vi "Example One Stage_Patrick_JKISM.vi"() -> ()   [LabVIEW 2019]
uses:
  <userlib>/LevyLab/Xeryon-Rotator/lvsrc/drivers/Class/Controller/Controller.lvclass
panel:
  out "Current State":string
  in  "Controller":refnum<class "Controller.lvclass">
  in  "STOP":bool
  out "Desired Position\n[selected units]":dbl
  out "Encoder position \n[selected units]":dbl
  in  "Tab Control":enum32{"Motion", "Settings"}(tab)
  in  "gotodesired":bool
  in  "Zero Output":bool
  in  "Go to Home":bool
  in  "Scan Right":bool
  in  "Scan Left":bool
  in  "Continue":bool
  in  "Stop":bool
  in  "Make Step Right":bool
  in  "Step Size \n[selected units]":dbl=1.0 format="%#.2f"
  in  "Make Step Left":bool
  in  "Desired Speed \n[1µm/s or 0,01deg /s]":dbl=10000.0 format="%#.2f"
  in  "Desired Position \n[selected units]":dbl format="%#.2f"
  in  "Find Index":bool
  in  "Reset":bool
  out "error out":errorcluster
  in  "Working Units":string(combo)="1000000,0"
  out "StatusBits":T1
  out "Status Info":T2
  in  "Axis Resolution":string(combo)="3.49065850399"
  in  "Axis Letter":string="X"
  in  "Baudrate":dbl=9600.0
  in  "COM Port":refnum<visa-resource-name>="COM4"
  out "Waveform Chart":T3(graph)
  in  "STOP PROGRAM":bool
  # "Visualization"
  # "Extra information"
  # "READ ME FIRST"
  # "Configuration"
  # "Stage 1"
  # "Driver 1"
  # "Stage 1"
  # "How to run:"
  # "BEFORE RUNNING:"
  # "1, Select COM Port"
  # "2. Select baudrate"
  # "3. For each axis:"
  # "3.1 Specify correct axis name (1 letter)"
  # "3.2 Specify correct resolution"
  # "4. Run VI"
  # "WHEN RUNNING, YOU HAVE TO FIRST PUSH \"FIND INDEX\" FOR EACH STAGE.\nThe stages will start moving and find its position. After that you can control the stages"
  # "NOTES: Do this only the first time"
  # "3.49065850399"
  # "1. Replace the settings_default.txt file with\nthe file we provided on a USB stick."
  # "2.    Make sure there are no comments in the\nsettings_default.txt file. ONLY lines like: \"X:DPOS=100\" so NO \"%\" in front or at the end of the line."
  # "Position Information"
  # "STOP BUTTON"
  # "3.  In your settings_default.txt file:\nEvery line that contains SSPD or MSPD: multiply that value with:\n - 1000 for a lineair stage \n - 100 for a rotating stage"
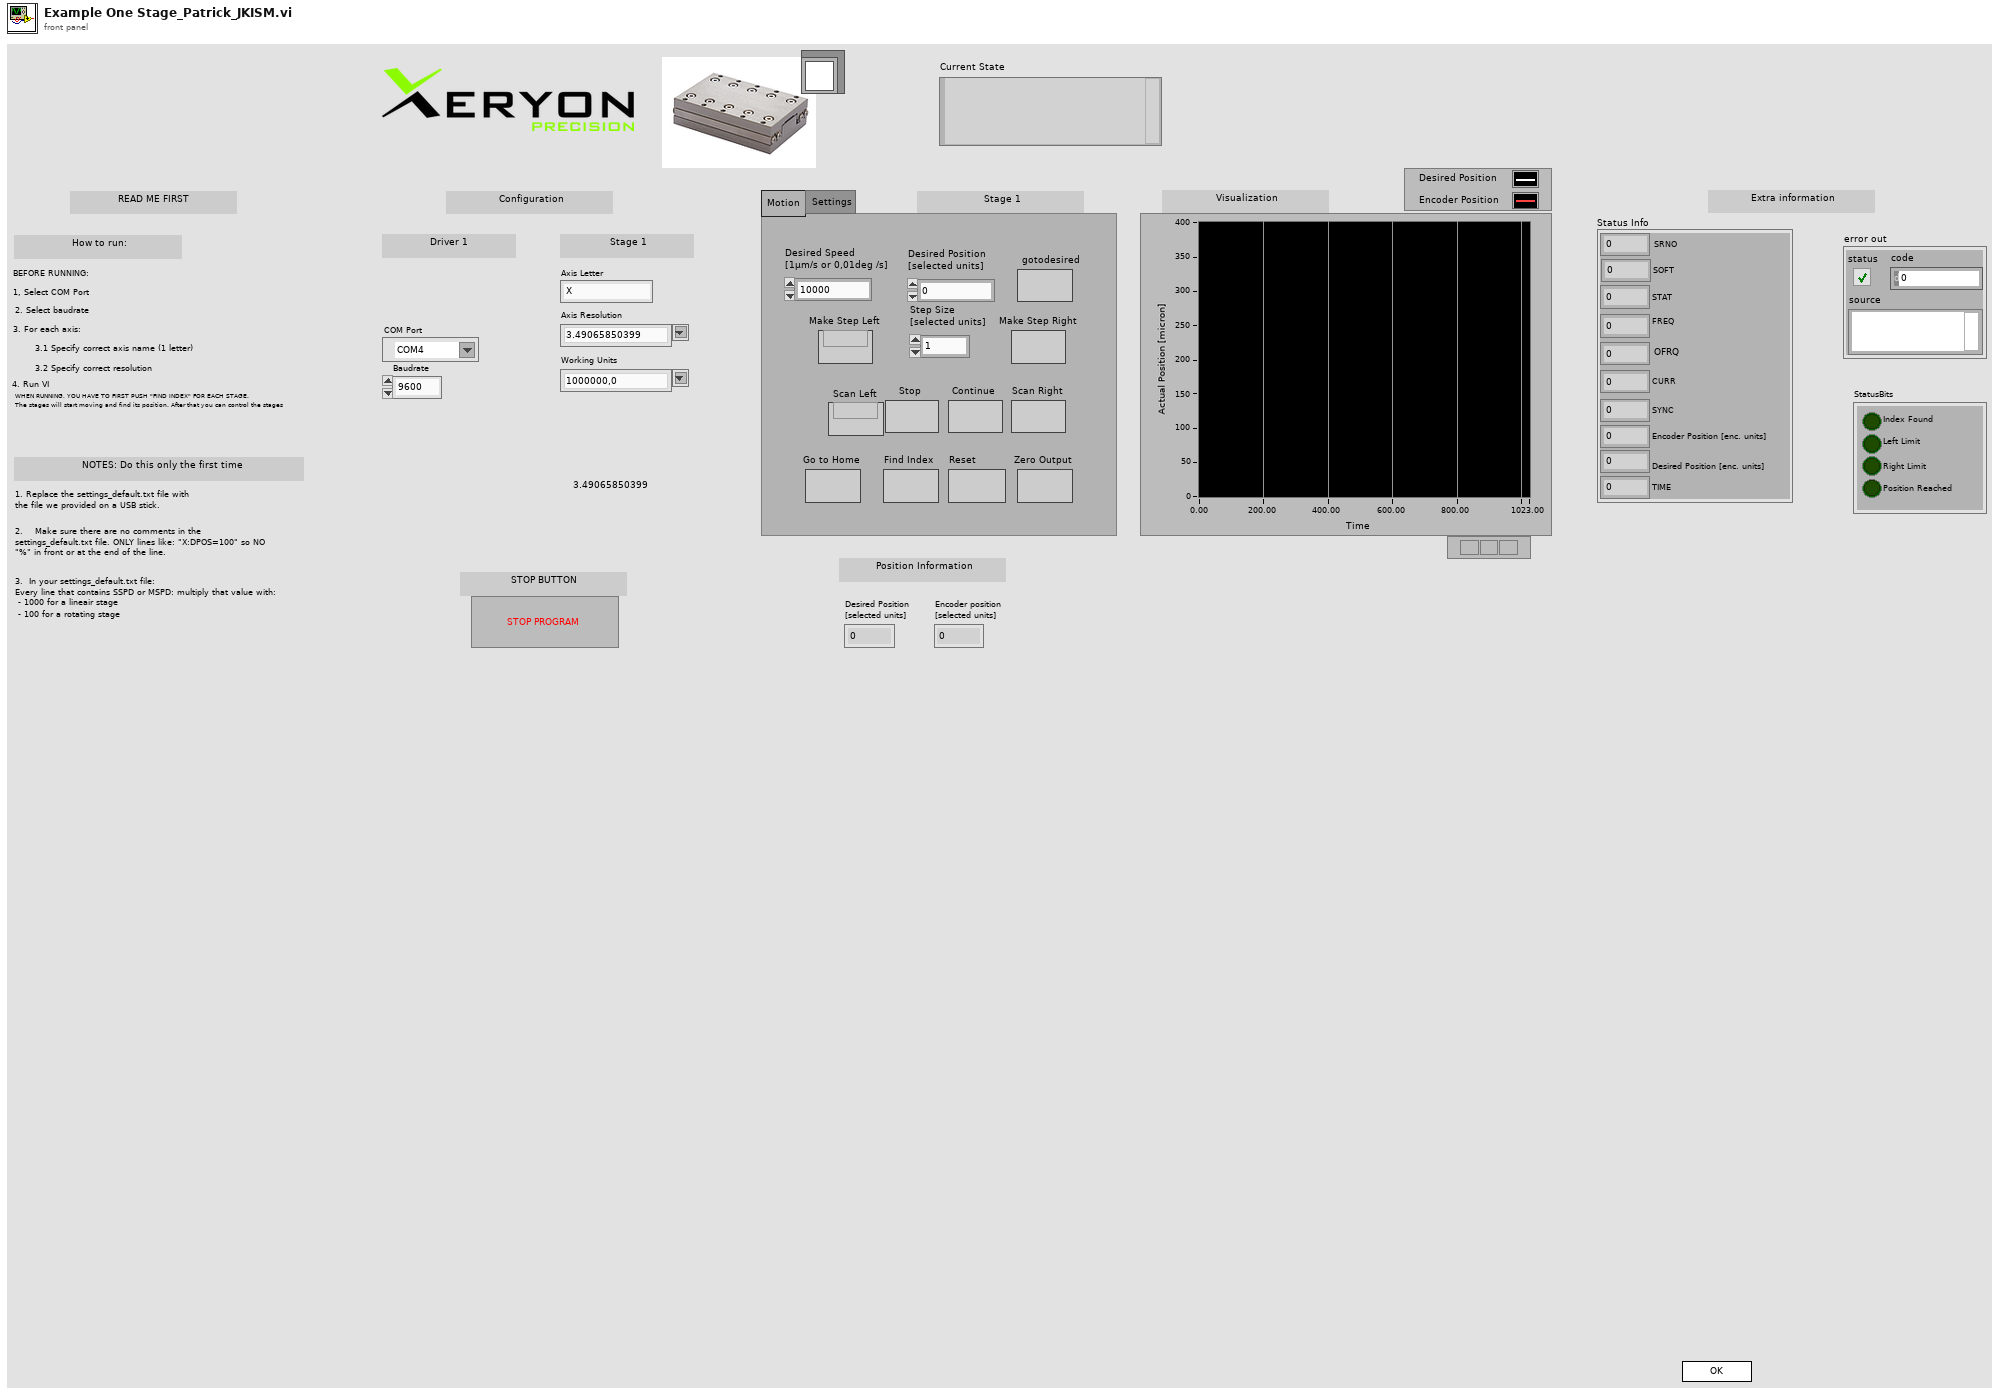
[diagram p1: front panel]
types:
  T1 = cluster{"Index Found":bool, "Left Limit":bool, "Right Limit":bool, "Position Reached":bool}
  T2 = cluster{"SRNO":dbl, "SOFT":dbl, "STAT":dbl, "FREQ":dbl, "OFRQ":dbl, "CURR":dbl, "SYNC":dbl, "Encoder Position [enc. units]":dbl, "Desired Position [enc. units]":dbl, "TIME":dbl}
  T3 = cluster{"DPOS In Current Units":dbl, "EPOS In Current Units":dbl}
  T4 = enum32{"Invalid", "Standard", "Closed", "Hidden", "Minimized", "Maximized"}
  T5 = enum32{"invalid app kind", "Development System", "Run Time System", "Student Edition", "Embedded LabVIEW", "Evaluation", "Custom"}
  T6 = cluster{"Core":cluster{"Current VI Reference":refnum<vi>, "Close Panel on Exit?":bool}, "Controller":refnum<class "Controller.lvclass">, "Axis Letter":string}
  T7 = cluster{"Current VI Reference":refnum<vi>, "Close Panel on Exit?":bool}
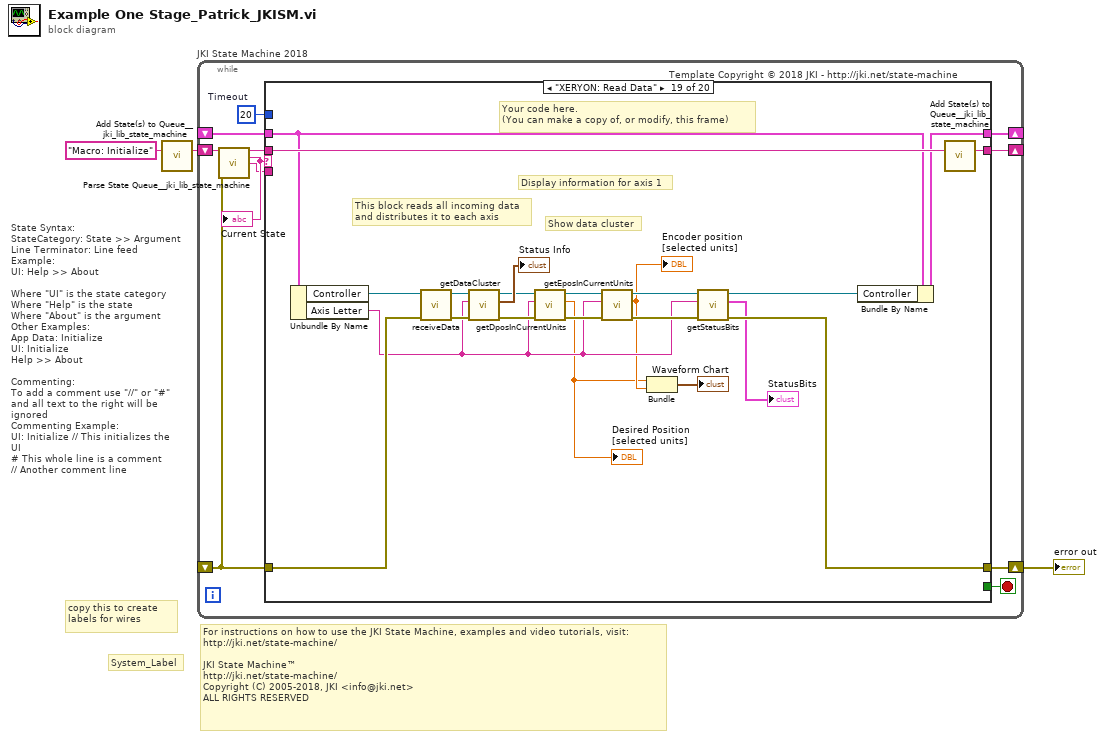
[diagram p0: block diagram]
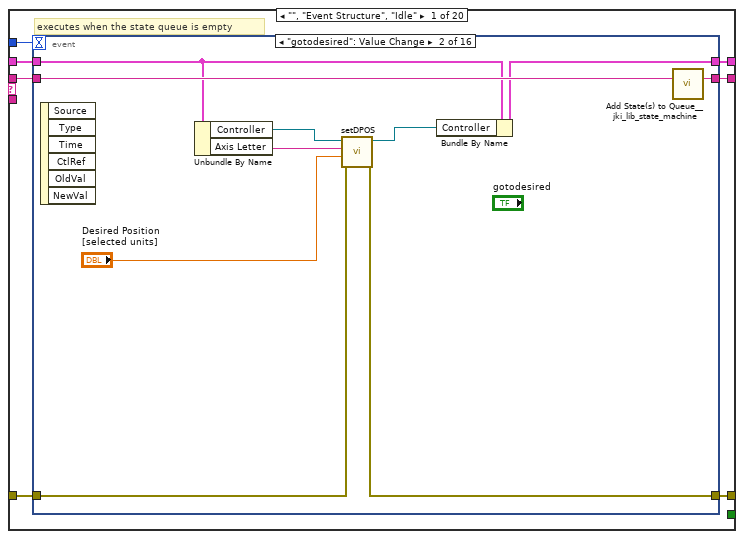
[diagram p2: hidden frame]
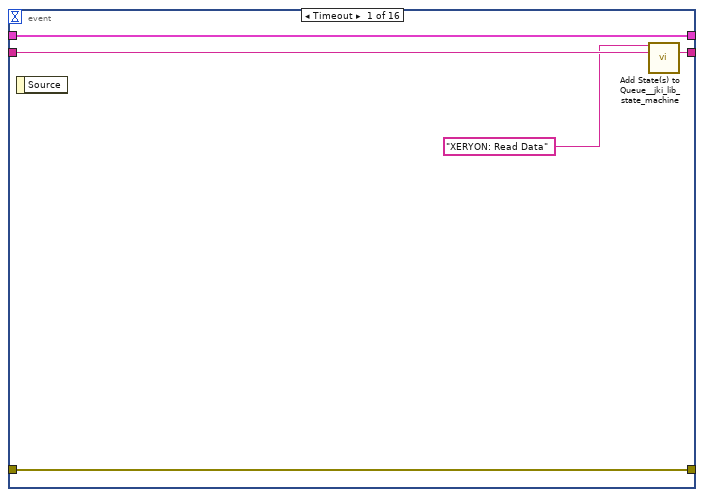
[diagram p3: hidden frame]
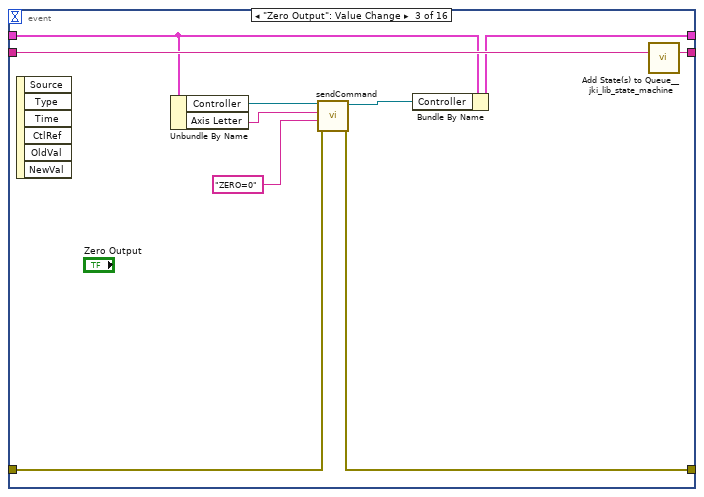
[diagram p4: hidden frame]
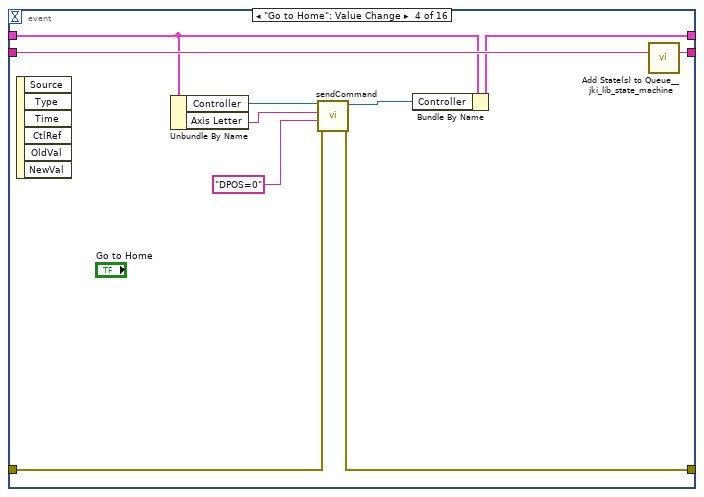
[diagram p5: hidden frame]
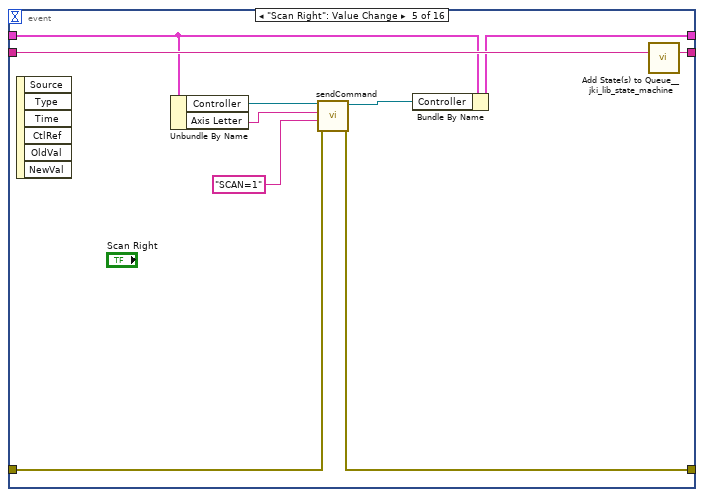
[diagram p6: hidden frame]
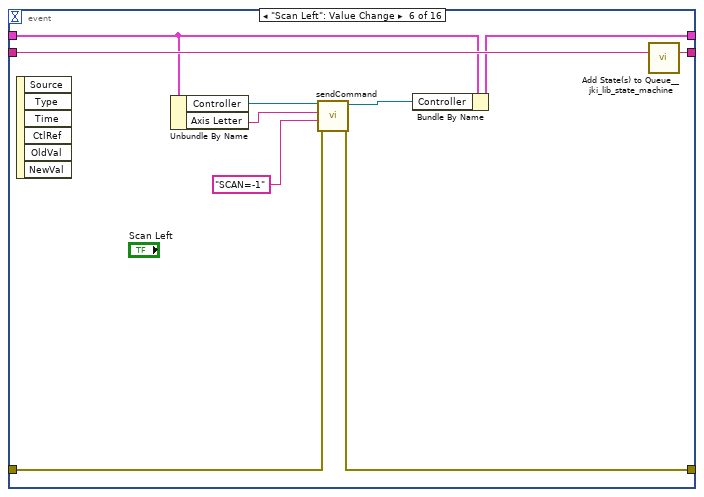
[diagram p7: hidden frame]
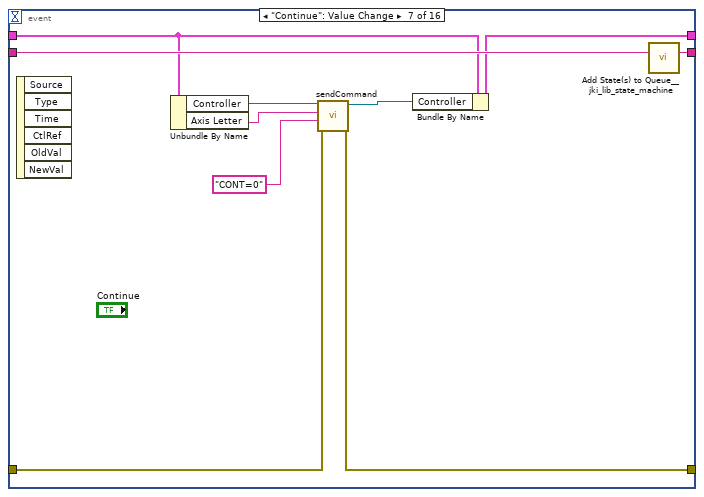
[diagram p8: hidden frame]
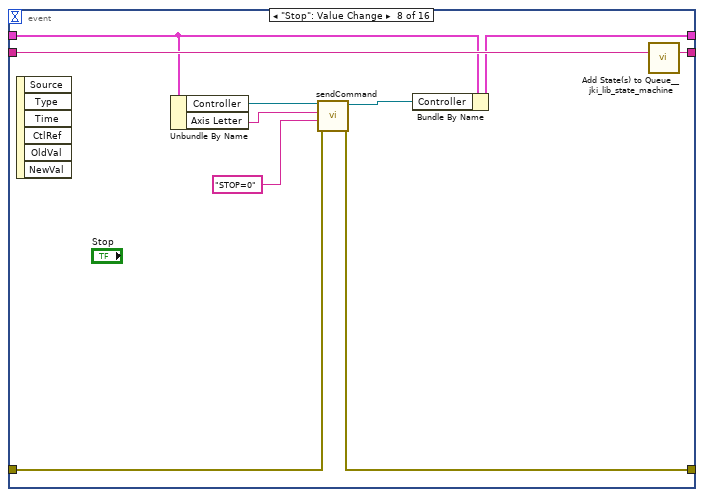
[diagram p9: hidden frame]
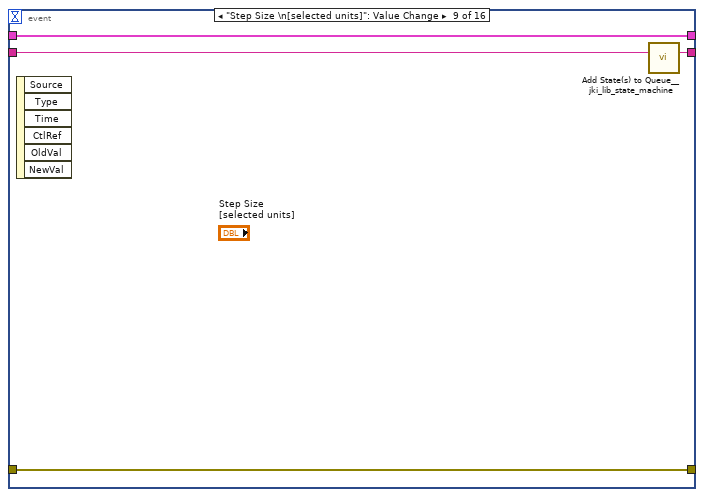
[diagram p10: hidden frame]
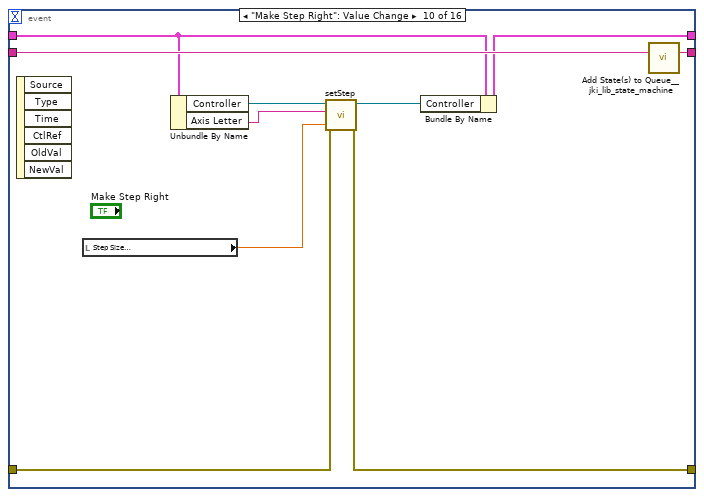
[diagram p11: hidden frame]
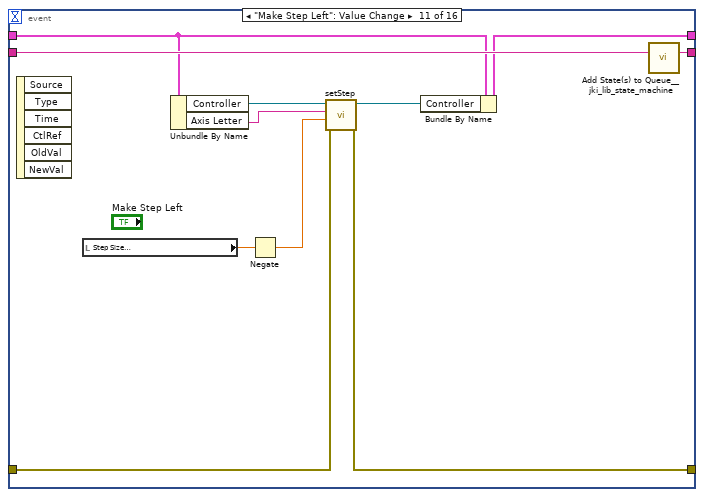
[diagram p12: hidden frame]
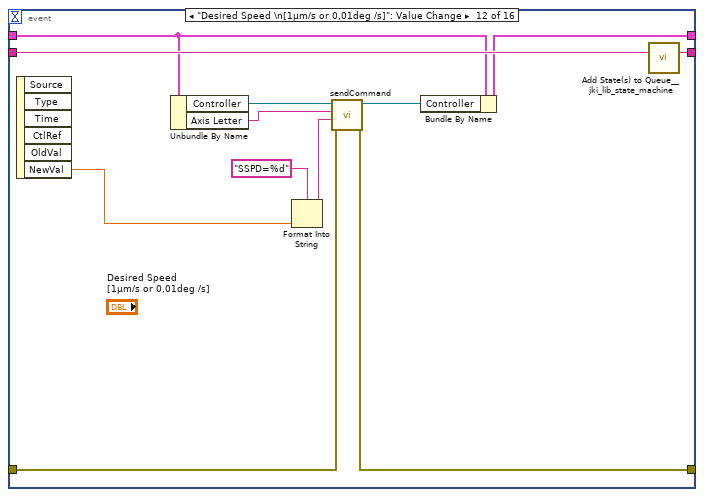
[diagram p13: hidden frame]
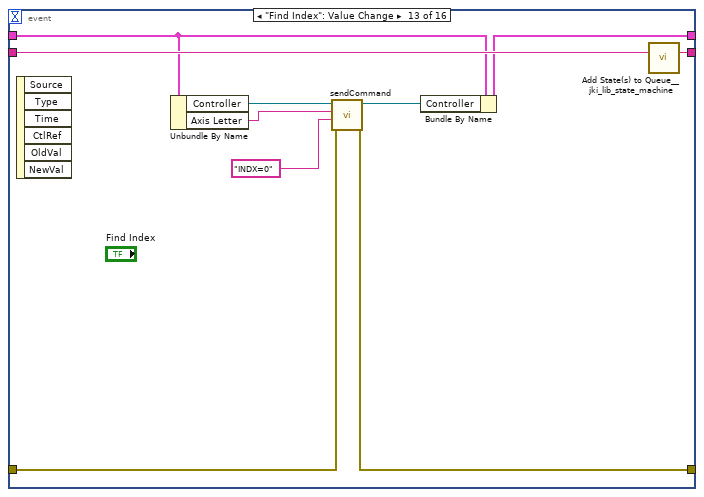
[diagram p14: hidden frame]
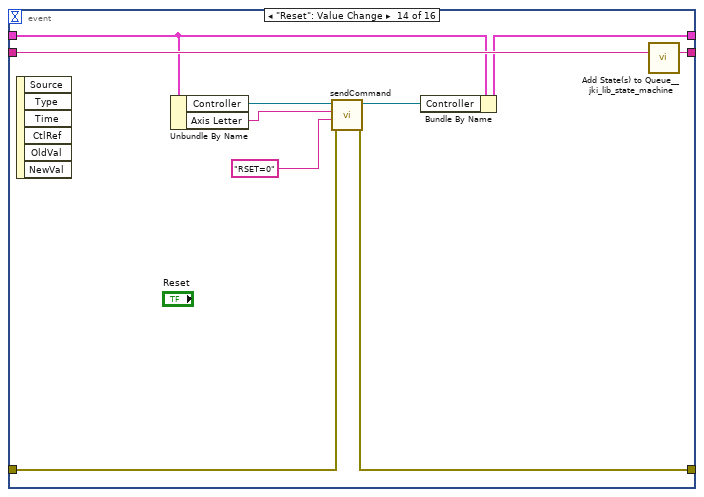
[diagram p15: hidden frame]
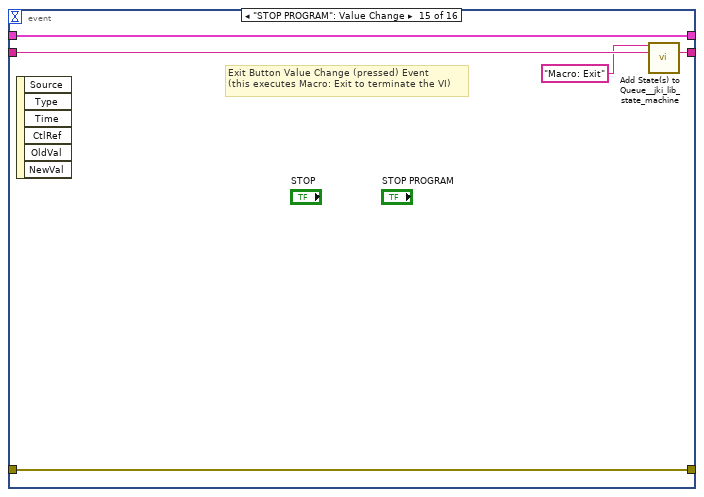
[diagram p16: hidden frame]
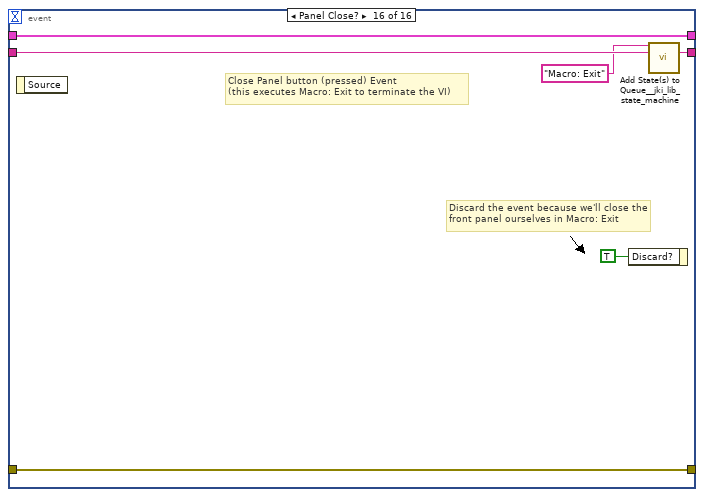
[diagram p17: hidden frame]
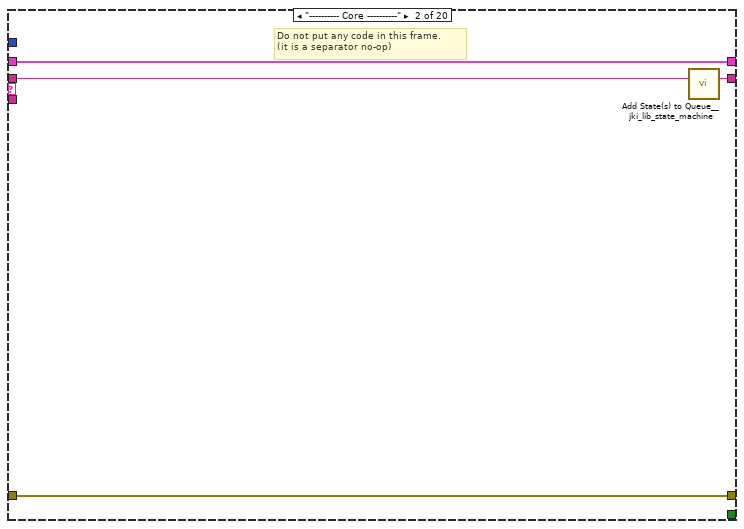
[diagram p18: hidden frame]
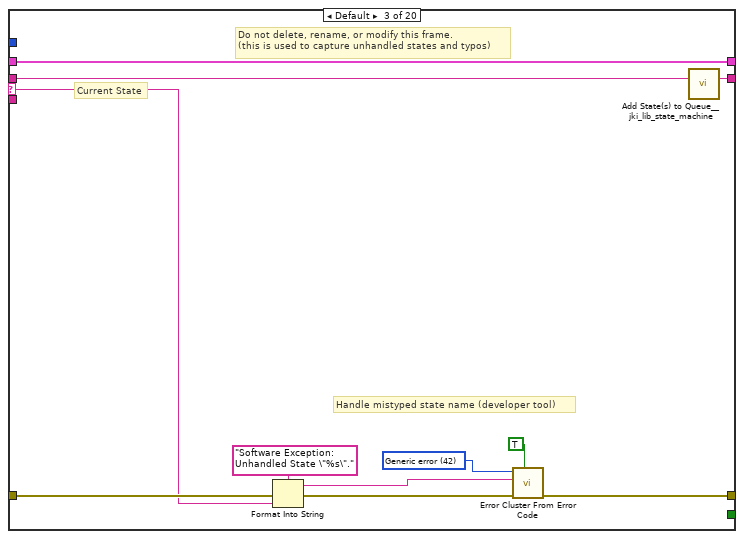
[diagram p19: hidden frame]
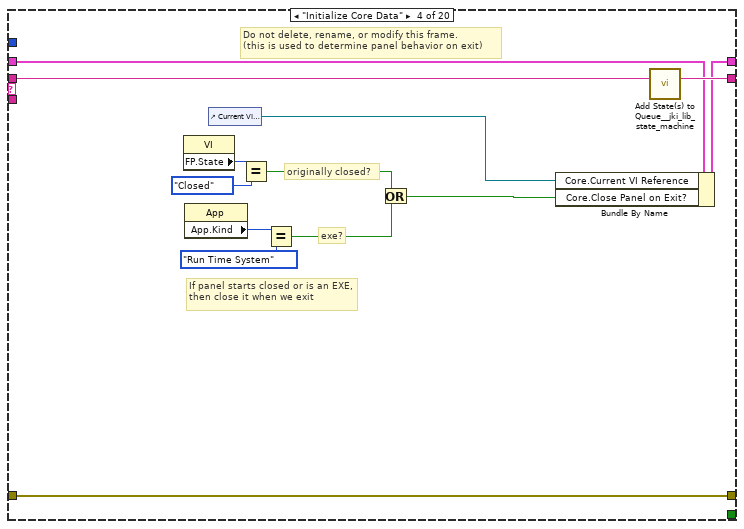
[diagram p20: hidden frame]
diagram:
  # "For instructions on how to use the JKI State Machine, examples and video tutorials, visit:\nhttp://jki.net/state-machine/\n\nJKI State Machine™\nhttp://jki.net/state-machine/\nCopyright (C) 2005-2018, JKI <info@jki.net>\nALL RIGHTS RESERVED"
  # "State Syntax:\nStateCategory: State >> Argument\nLine Terminator: Line feed\nExample:\nUI: Help >> About\n\nWhere \"UI\" is the state category\nWhere \"Help\" is the state\nWhere \"About\" is the argument\nOther Examples:\nApp Data: Initialize\nUI: Initialize\nHelp >> About\n\nCommenting:\nTo add a comment use \"//\" or \"#\" and all text to the right will be ignored\nCommenting Example:\nUI: Initialize // This initializes the UI\n# This whole line is a comment\n// Another comment line"
  # "copy this to create labels for wires"
  # "System_Label"
  n1 = call <vilib>:"Add State(s) to Queue__jki_lib_state_machine.vi"("State(s) in (\"\")"="Macro: Initialize") -> ("States Out"=w3:string)  [unwired: 14 in]
  n2 = while "JKI State Machine 2018" {
    shift-right: [w7] -> _
    shift-left: _ -> [w6]
    shift-right: [w10] -> w1
    shift-left: _ -> [w4]
    shift-right: [w9] -> _
    shift-left: w3 -> [w11]
    stop <- w8 stop-if-true
    w5 = 20  # Timeout
    # "Template Copyright © 2018 JKI - http://jki.net/state-machine"
    n3 = call <vilib>:"Parse State Queue__jki_lib_state_machine.vi"("State Queue"=w11, "Error In (no error)"=w4) -> ("Remaining States"=w13:string, "Current State"=w14:string, "Arguments"=w12:string)  [unwired: 11 in]
    "Current State" <- w14
    n4 = case shown="\"XERYON: Read Data\"" w14 {
      selector: w14 -> [_ _ w169 _ _ _ _ _ _ _ _ _ _ _ _ _ _ _ _ _]
      tunnel: w13 -> [w21 w168 w173 w192 w198 w203 w207 w214 w220 w224 w228 w234 w245 w314 w319 w330 w334 w351 w373 w379]
      tunnel: w12 -> [_ _ _ _ _ _ _ _ _ _ _ w229 w239 _ _ _ _ _ _ _]
      tunnel: w6 -> [w19 w165 w171 w185 w195 w201 w204 _ w215 w221 w226 w232 w241 w311 w316 w327 w331 w338 w356 w377]
      tunnel: [w18 w166 w175 w189 errorcluster {"status"=FALSE, "code"=0, "source"=""} ("error out") w200 w205 w211 w216 w222 w225 w230 w242 w312 w317 w328 w332 w336 w360 w375] -> w10
      tunnel: w4 -> [w17 w166 w174 w189 w194 w200 w205 w211 w217 w222 w225 w231 w243 w312 w317 w328 w332 w335 w359 w374]
      tunnel: [w20 w167 w172 w191 w197 w202 w206 w213 w219 w223 w227 w233 w244 w313 w318 w329 w333 w350 w372 w378] -> w9
      tunnel: [_ _ _ _ _ TRUE _ _ _ _ _ _ _ _ _ _ _ _ _ _] -> w8
      tunnel: [w16 w165 w171 w190 w195 w201 w204 w212 w215 w221 w226 w232 w241 w311 w316 w327 w331 w349 w357 w377] -> w7
      tunnel: w5 -> [w15 _ _ _ _ _ _ _ _ _ _ _ _ _ _ _ _ _ _ _]
      frame "", "Event Structure", "Idle" {
        # "executes when the state queue is empty"
        n5 = event shown="[1] \"gotodesired\": Value Change" {
          selector: _ -> [_ _ _ _ _ _ _ _ _ _ _ _ _ _ _ _]
          dyn-events: _ -> [_ _ _ _ _ _ _ _ _ _ _ _ _ _ _ _]
          timeout: w15 -> [_ _ _ _ _ _ _ _ _ _ _ _ _ _ _ _]
          tunnel: w21 -> [w26 w36 w46 w56 w66 w76 w86 w96 w100 w110 w121 w133 w143 w153 w158 w164]
          tunnel: [w25 w35 w45 w55 w65 w75 w85 w95 w99 w109 w120 w132 w142 w152 w157 w163] -> w20
          tunnel: w19 -> [w23 w30 w43 w53 w63 w73 w83 w93 w98 w107 w118 w130 w140 w150 w155 w161]
          tunnel: [w24 w29 w37 w47 w57 w67 w77 w87 w97 w101 w112 w122 w135 w145 w156 w162] -> w18
          tunnel: w17 -> [w24 w28 w38 w48 w58 w68 w78 w88 w97 w102 w113 w123 w136 w146 w156 w162]
          tunnel: [w23 w31 w44 w54 w64 w74 w84 w94 w98 w108 w119 w131 w141 w151 w155 w161] -> w16
          event Timeout {
            n6 = event-data() -> ()  [unwired: 1 in, 1 out]
            n7 = call <vilib>:"Add State(s) to Queue__jki_lib_state_machine.vi"("State(s) in Front (\"\")"="XERYON: Read Data" ("State(s) in Front (\"\")"), "State(s) in (\"\")"=w26) -> ("States Out"=w25:string)  [unwired: 13 in]
          }
          event "gotodesired": Value Change {
            n8 = event-data() -> ()  [unwired: 1 in, 6 out]
            n9 = Unbundle By Name(w30) -> ("Controller"=w33:refnum<class "Controller.lvclass">, "Axis Letter"=w34:string)
            n10 = call-dynamic "setDPOS.vi"("error in (no error)"=w28, "DPOS In Current Units"="Desired Position \n[selected units]", "Axis Letter"=w34, "Controller in"=w33) -> ("error out"=w29:errorcluster, "Controller out"=w32:refnum<class "Controller.lvclass">)  [unwired: 6 in]
            n11 = Bundle By Name(cluster=w30, "Controller"=w32) -> (w31:T6)
            n12 = call <vilib>:"Add State(s) to Queue__jki_lib_state_machine.vi"("State(s) in (\"\")"=w36) -> ("States Out"=w35:string)  [unwired: 14 in]
          }
          event "Zero Output": Value Change {
            n13 = event-data() -> ()  [unwired: 1 in, 6 out]
            n14 = Unbundle By Name(w43) -> ("Controller"=w41:refnum<class "Controller.lvclass">, "Axis Letter"=w40:string)
            n15 = call-dynamic "sendCommand.vi"("error in (no error)"=w38, "Command"="ZERO=0", "Axis Letter"=w40, "Controller in"=w41) -> ("error out"=w37:errorcluster, "Controller out"=w39:refnum<class "Controller.lvclass">)  [unwired: 6 in]
            n16 = Bundle By Name(cluster=w43, "Controller"=w39) -> (w44:T6)
            n17 = call <vilib>:"Add State(s) to Queue__jki_lib_state_machine.vi"("State(s) in (\"\")"=w46) -> ("States Out"=w45:string)  [unwired: 14 in]
          }
          event "Go to Home": Value Change {
            n18 = event-data() -> ()  [unwired: 1 in, 6 out]
            n19 = Unbundle By Name(w53) -> ("Controller"=w51:refnum<class "Controller.lvclass">, "Axis Letter"=w50:string)
            n20 = call-dynamic "sendCommand.vi"("error in (no error)"=w48, "Command"="DPOS=0", "Axis Letter"=w50, "Controller in"=w51) -> ("error out"=w47:errorcluster, "Controller out"=w49:refnum<class "Controller.lvclass">)  [unwired: 6 in]
            n21 = Bundle By Name(cluster=w53, "Controller"=w49) -> (w54:T6)
            n22 = call <vilib>:"Add State(s) to Queue__jki_lib_state_machine.vi"("State(s) in (\"\")"=w56) -> ("States Out"=w55:string)  [unwired: 14 in]
          }
          event "Scan Right": Value Change {
            n23 = event-data() -> ()  [unwired: 1 in, 6 out]
            n24 = Unbundle By Name(w63) -> ("Controller"=w61:refnum<class "Controller.lvclass">, "Axis Letter"=w60:string)
            n25 = call-dynamic "sendCommand.vi"("error in (no error)"=w58, "Command"="SCAN=1", "Axis Letter"=w60, "Controller in"=w61) -> ("error out"=w57:errorcluster, "Controller out"=w59:refnum<class "Controller.lvclass">)  [unwired: 6 in]
            n26 = Bundle By Name(cluster=w63, "Controller"=w59) -> (w64:T6)
            n27 = call <vilib>:"Add State(s) to Queue__jki_lib_state_machine.vi"("State(s) in (\"\")"=w66) -> ("States Out"=w65:string)  [unwired: 14 in]
          }
          event "Scan Left": Value Change {
            n28 = event-data() -> ()  [unwired: 1 in, 6 out]
            n29 = Unbundle By Name(w73) -> ("Controller"=w71:refnum<class "Controller.lvclass">, "Axis Letter"=w70:string)
            n30 = call-dynamic "sendCommand.vi"("error in (no error)"=w68, "Command"="SCAN=-1", "Axis Letter"=w70, "Controller in"=w71) -> ("error out"=w67:errorcluster, "Controller out"=w69:refnum<class "Controller.lvclass">)  [unwired: 6 in]
            n31 = Bundle By Name(cluster=w73, "Controller"=w69) -> (w74:T6)
            n32 = call <vilib>:"Add State(s) to Queue__jki_lib_state_machine.vi"("State(s) in (\"\")"=w76) -> ("States Out"=w75:string)  [unwired: 14 in]
          }
          event "Continue": Value Change {
            n33 = event-data() -> ()  [unwired: 1 in, 6 out]
            n34 = Unbundle By Name(w83) -> ("Controller"=w81:refnum<class "Controller.lvclass">, "Axis Letter"=w80:string)
            n35 = call-dynamic "sendCommand.vi"("error in (no error)"=w78, "Command"="CONT=0", "Axis Letter"=w80, "Controller in"=w81) -> ("error out"=w77:errorcluster, "Controller out"=w79:refnum<class "Controller.lvclass">)  [unwired: 6 in]
            n36 = Bundle By Name(cluster=w83, "Controller"=w79) -> (w84:T6)
            n37 = call <vilib>:"Add State(s) to Queue__jki_lib_state_machine.vi"("State(s) in (\"\")"=w86) -> ("States Out"=w85:string)  [unwired: 14 in]
          }
          event "Stop": Value Change {
            n38 = event-data() -> ()  [unwired: 1 in, 6 out]
            n39 = Unbundle By Name(w93) -> ("Controller"=w91:refnum<class "Controller.lvclass">, "Axis Letter"=w90:string)
            n40 = call-dynamic "sendCommand.vi"("error in (no error)"=w88, "Command"="STOP=0", "Axis Letter"=w90, "Controller in"=w91) -> ("error out"=w87:errorcluster, "Controller out"=w89:refnum<class "Controller.lvclass">)  [unwired: 6 in]
            n41 = Bundle By Name(cluster=w93, "Controller"=w89) -> (w94:T6)
            n42 = call <vilib>:"Add State(s) to Queue__jki_lib_state_machine.vi"("State(s) in (\"\")"=w96) -> ("States Out"=w95:string)  [unwired: 14 in]
          }
          event "Step Size \n[selected units]": Value Change {
            n43 = event-data() -> ()  [unwired: 1 in, 6 out]
            n44 = call <vilib>:"Add State(s) to Queue__jki_lib_state_machine.vi"("State(s) in (\"\")"=w100) -> ("States Out"=w99:string)  [unwired: 14 in]
          }
          event "Make Step Right": Value Change {
            n45 = event-data() -> ()  [unwired: 1 in, 6 out]
            n46 = local read "Step Size \n[selected units]"() -> (w103:dbl)
            n47 = Unbundle By Name(w107) -> ("Controller"=w106:refnum<class "Controller.lvclass">, "Axis Letter"=w104:string)
            n48 = call-dynamic "setStep.vi"("error in (no error)"=w102, "Step Value"=w103, "Axis Letter"=w104, "Controller in"=w106) -> ("error out"=w101:errorcluster, "Controller out"=w105:refnum<class "Controller.lvclass">)  [unwired: 6 in]
            n49 = Bundle By Name(cluster=w107, "Controller"=w105) -> (w108:T6)
            n50 = call <vilib>:"Add State(s) to Queue__jki_lib_state_machine.vi"("State(s) in (\"\")"=w110) -> ("States Out"=w109:string)  [unwired: 14 in]
          }
          event "Make Step Left": Value Change {
            n51 = event-data() -> ()  [unwired: 1 in, 6 out]
            n52 = local read "Step Size \n[selected units]"() -> (w114:dbl)
            n53 = Unbundle By Name(w118) -> ("Controller"=w117:refnum<class "Controller.lvclass">, "Axis Letter"=w115:string)
            n54 = Negate(x=w114) -> (-x=w111:dbl)
            n55 = call-dynamic "setStep.vi"("error in (no error)"=w113, "Step Value"=w111, "Axis Letter"=w115, "Controller in"=w117) -> ("error out"=w112:errorcluster, "Controller out"=w116:refnum<class "Controller.lvclass">)  [unwired: 6 in]
            n56 = Bundle By Name(cluster=w118, "Controller"=w116) -> (w119:T6)
            n57 = call <vilib>:"Add State(s) to Queue__jki_lib_state_machine.vi"("State(s) in (\"\")"=w121) -> ("States Out"=w120:string)  [unwired: 14 in]
          }
          event "Desired Speed \n[1µm/s or 0,01deg /s]": Value Change {
            n58 = event-data() -> ("NewVal"=w124:dbl)  [unwired: 1 in, 5 out]
            n59 = Unbundle By Name(w130) -> ("Controller"=w127:refnum<class "Controller.lvclass">, "Axis Letter"=w125:string)
            n60 = Format Into String(format string="SSPD=%d", w124) -> (resulting string=w129:string)  [unwired: 2 in, 1 out]
            n61 = call-dynamic "sendCommand.vi"("error in (no error)"=w123, "Command"=w129, "Axis Letter"=w125, "Controller in"=w127) -> ("error out"=w122:errorcluster, "Controller out"=w126:refnum<class "Controller.lvclass">)  [unwired: 6 in]
            n62 = Bundle By Name(cluster=w130, "Controller"=w126) -> (w131:T6)
            n63 = call <vilib>:"Add State(s) to Queue__jki_lib_state_machine.vi"("State(s) in (\"\")"=w133) -> ("States Out"=w132:string)  [unwired: 14 in]
          }
          event "Find Index": Value Change {
            n64 = event-data() -> ()  [unwired: 1 in, 6 out]
            n65 = Unbundle By Name(w140) -> ("Controller"=w139:refnum<class "Controller.lvclass">, "Axis Letter"=w137:string)
            n66 = call-dynamic "sendCommand.vi"("error in (no error)"=w136, "Command"="INDX=0", "Axis Letter"=w137, "Controller in"=w139) -> ("error out"=w135:errorcluster, "Controller out"=w138:refnum<class "Controller.lvclass">)  [unwired: 6 in]
            n67 = Bundle By Name(cluster=w140, "Controller"=w138) -> (w141:T6)
            n68 = call <vilib>:"Add State(s) to Queue__jki_lib_state_machine.vi"("State(s) in (\"\")"=w143) -> ("States Out"=w142:string)  [unwired: 14 in]
          }
          event "Reset": Value Change {
            n69 = event-data() -> ()  [unwired: 1 in, 6 out]
            n70 = Unbundle By Name(w150) -> ("Controller"=w149:refnum<class "Controller.lvclass">, "Axis Letter"=w147:string)
            n71 = call-dynamic "sendCommand.vi"("error in (no error)"=w146, "Command"="RSET=0", "Axis Letter"=w147, "Controller in"=w149) -> ("error out"=w145:errorcluster, "Controller out"=w148:refnum<class "Controller.lvclass">)  [unwired: 6 in]
            n72 = Bundle By Name(cluster=w150, "Controller"=w148) -> (w151:T6)
            n73 = call <vilib>:"Add State(s) to Queue__jki_lib_state_machine.vi"("State(s) in (\"\")"=w153) -> ("States Out"=w152:string)  [unwired: 14 in]
          }
          event "STOP PROGRAM": Value Change {
            # "Exit Button Value Change (pressed) Event\n(this executes Macro: Exit to terminate the VI)"
            n74 = event-data() -> ()  [unwired: 1 in, 6 out]
            n75 = call <vilib>:"Add State(s) to Queue__jki_lib_state_machine.vi"("State(s) in Front (\"\")"="Macro: Exit", "State(s) in (\"\")"=w158) -> ("States Out"=w157:string)  [unwired: 13 in]
          }
          event Panel Close? {
            # "Discard the event because we'll close the front panel ourselves in Macro: Exit"
            # "Close Panel button (pressed) Event\n(this executes Macro: Exit to terminate the VI)"
            n76 = event-data() -> ()  [unwired: 1 in, 1 out]
            n77 = event-data("Discard?"=TRUE) -> ()  [unwired: 1 in, 1 out]
            n78 = call <vilib>:"Add State(s) to Queue__jki_lib_state_machine.vi"("State(s) in Front (\"\")"="Macro: Exit", "State(s) in (\"\")"=w164) -> ("States Out"=w163:string)  [unwired: 13 in]
          }
        }
      }
      frame "---------- Core ----------" {
        # "Do not put any code in this frame.\n(it is a separator no-op)"
        n79 = call <vilib>:"Add State(s) to Queue__jki_lib_state_machine.vi"("State(s) in (\"\")"=w168) -> ("States Out"=w167:string)  [unwired: 14 in]
      }
      frame Default {
        w178 = 42 items=["No error", "Argument error", "Memory is full", "Out of zone", "End of file", "File already open", "Generic file I/O error", "File not found", "File permission error", "Disk is full", "Duplicate path", "Too many files open", "System feature not enabled", "Resource file not found", "Cannot add resource", "Resource not found", "Image not found", "Image memory error", "Pen does not exist", "Config type invalid", "Config token not found", "Config parse error", "Config memory error", "Bad external code format", "Bad external code offset", "External code not present", "Null window", "Destroy window error", "Null menu", "Print aborted", "Bad print record", "Print driver error", "Windows error during printing", "Memory error during printing", "Print dialog error", "Generic print error", "Invalid device refnum", "Device not found", "Device parameter error", "Device unit error", "Cannot open device", "Device call aborted", "Generic error", "Cancelled by user", "Object ID too low", "Object ID too high", "Object not in heap", "Unknown heap", "Unknown object (invalid DefProc)", "Unknown object (DefProc not in table)", "Message out of range", "Invalid (null) method", "Unknown message", "Manager call not supported", "Bad address", "Network operation in progress", "Network operation timed out", "Connection is busy", "Network attribute not supported", "Network error", "Address in use", "System out of memory", "Connection aborted", "Connection refused", "Not connected", "Already connected", "Connection closed", "Initialization error (interapplication manager)", "Bad occurrence", "Wait on unbound occurrence handler", "Occurrence queue overflow", "Datalog type conflict", "Unused", "Unrecognized type (interapplication manager)", "Memory corrupt", "Failed to make temporary DLL", "Old CIN version", "Drag socket not found", "Failed to load drop-object", "Failed to register OLE object", "Failed to release OLE object", "Format specifier type mismatch", "Unknown format specifier", "Too few format specifiers", "Too many format specifiers", "Scan failed", "Newer CIN version", "Error converting to variant", "Runtime menu error", "Password tampered", "Variant attribute not found", "Incompatible variant data type", "Event data is not available", "Event Store is not present", "Occurrence is not found", "Event Queue is not created", "Event info is not available", "Refnum passed is NULL", "Error retrieving Class GUID", "Error retrieving CoClass GUID", "Error retrieving TypeLib GUID.", "Bad built application magic bytes.", "Specific driver is different from the specific driver associated with the Logical Name.", "There is no session opened to the class driver.", "Max Error", "MAX - Error with config objects", "MAX - Error loading configuration", "MAX - Group not supported"]
        # "Current State"
        # "Do not delete, rename, or modify this frame.\n(this is used to capture unhandled states and typos)"
        # "Handle mistyped state name (developer tool)"
        n80 = Format Into String(format string="Software Exception: Unhandled State \"%s\"." ("message"), error in=w174, w169) -> (resulting string=w177:string, error out=w176:errorcluster)  [unwired: 1 in]
        n81 = call <vilib>:"Error Cluster From Error Code.vi"("show call chain? (False)"=TRUE, "error in (no error)"=w176, "error message (\"\")"=w177, "error code (0)"=w178) -> ("error out"=w175:errorcluster)  [unwired: 5 in]
        n82 = call <vilib>:"Add State(s) to Queue__jki_lib_state_machine.vi"("State(s) in (\"\")"=w173) -> ("States Out"=w172:string)  [unwired: 14 in]
      }
      frame "Initialize Core Data" {
        # "Do not delete, rename, or modify this frame.\n(this is used to determine panel behavior on exit)"
        # "originally closed?"
        # "exe?"
        # "If panel starts closed or is an EXE, then close it when we exit"
        n83 = property class="VI"() -> ("FP.State"=w182:T4)  [unwired: 2 in, 2 out]
        n84 = property class="App"() -> ("App.Kind"=w188:T5)  [unwired: 2 in, 2 out]
        n85 = control-ref of="Current VI Reference"() -> (w183:refnum<vi>)
        n86 = Equal?(x=w182, y=T4."Closed" ("Front Panel Window:State")) -> (x = y?=w180:bool)
        n87 = Equal?(x=w188, y=T5."Run Time System" ("Application:Kind")) -> (x = y?=w186:bool)
        n88 = Or(x=w180, y=w186) -> (x .or. y?=w184:bool)
        n89 = Bundle By Name(cluster=w185, "Core.Current VI Reference"=w183, "Core.Close Panel on Exit?"=w184) -> (w190:T6)
        n90 = call <vilib>:"Add State(s) to Queue__jki_lib_state_machine.vi"("State(s) in (\"\")"=w192) -> ("States Out"=w191:string)  [unwired: 14 in]
      }
      frame "Error Handler" {
        # "Unhandled Error -- Display it"
        # "Handle any errors here.\nYou can also output any states to clean-up after errors occur"
        # "Clear error"
        n91 = call <vilib>:"General Error Handler.vi"("error in (no error)"=w194) -> ()  [unwired: 10 in, 5 out]
        n92 = call <vilib>:"Add State(s) to Queue__jki_lib_state_machine.vi"("State(s) in Front (\"\")"="/* Post Error States", "State(s) in (\"\")"=w198) -> ("States Out"=w197:string)  [unwired: 13 in]
      }
      frame "Exit" {
        # "Do not put any code in this frame.\n(No errors that occur here will be handled.)"
        n93 = call <vilib>:"Add State(s) to Queue__jki_lib_state_machine.vi"("State(s) in (\"\")"=w203) -> ("States Out"=w202:string)  [unwired: 14 in]
      }
      frame "---------- Data ----------" {
        # "Do not put any code in this frame.\n(It is a separator no-op. You can make a copy of this frame to create a new Data frame)"
        n94 = call <vilib>:"Add State(s) to Queue__jki_lib_state_machine.vi"("State(s) in (\"\")"=w207) -> ("States Out"=w206:string)  [unwired: 14 in]
      }
      frame "Data: Initialize" {
        w208 = "X"  # Axis Letter
        w210 = T7 {"Current VI Reference"=refnum, "Close Panel on Exit?"=FALSE}  # Core
        # "Initialize the shift-register data, here.\n(data names are defined by what you wire into the bundle function)"
        n95 = Bundle("Core"=w210, "Controller"="Controller", "Axis Letter"=w208) -> (w212:T6)  [unwired: 1 in]
        n96 = call <vilib>:"Add State(s) to Queue__jki_lib_state_machine.vi"("State(s) in (\"\")"=w214) -> ("States Out"=w213:string)  [unwired: 14 in]
      }
      frame "Data: Cleanup" {
        # "Cleanup any data and references, here.\n(this is called automatically, by the Macro: Exit)"
        n97 = Unbundle By Name(w215) -> ("Core.Current VI Reference"=w218:refnum<vi>)
        n98 = Close Reference(reference=w218, error in (no error)=w217) -> (error out=w216:errorcluster)
        n99 = call <vilib>:"Add State(s) to Queue__jki_lib_state_machine.vi"("State(s) in (\"\")"=w220) -> ("States Out"=w219:string)  [unwired: 14 in]
      }
      frame "---------- UI ----------" {
        # "Do not put any code in this frame.\n(It is a separator no-op. You can make a copy of this frame to create a new UI frame)"
        n100 = call <vilib>:"Add State(s) to Queue__jki_lib_state_machine.vi"("State(s) in (\"\")"=w224) -> ("States Out"=w223:string)  [unwired: 14 in]
      }
      frame "UI: Initialize" {
        # "Initialize the User Interface, here.\n(this is called automatically, by the Macro: Init)"
        n101 = call <vilib>:"Add State(s) to Queue__jki_lib_state_machine.vi"("State(s) in (\"\")"=w228) -> ("States Out"=w227:string)  [unwired: 14 in]
      }
      frame "UI: Cursor Set" {
        # "Argument"
        # "Set and Unset Cursor Busy.\n(Usage: \"UI: Cursor Set >> Busy|Idle\")"
        n102 = case shown="\"Idle\", Default" w229 {
          tunnel: w231 -> [w236 w238]
          tunnel: [w235 w237] -> w230
          frame "Idle", Default {
            n103 = call <vilib>:"Unset Busy.vi"("error in (no error)"=w236) -> ("error out"=w235:errorcluster)  [unwired: 10 in]
          }
          frame "Busy" {
            n104 = call <vilib>:"Set Busy.vi"("error in (no error)"=w238) -> ("error out"=w237:errorcluster)  [unwired: 9 in, 1 out]
          }
        }
        n105 = call <vilib>:"Add State(s) to Queue__jki_lib_state_machine.vi"("State(s) in (\"\")"=w234) -> ("States Out"=w233:string)  [unwired: 14 in]
      }
      frame "UI: Front Panel State" {
        # "Argument"
        # "Set Front Panel Open or Closed\n(Usage: \"UI: Front Panel State >> Open|Close\")"
        n106 = Unbundle By Name(w241) -> ("Core.Current VI Reference"=w240:refnum<vi>)
        n107 = case shown="\"Minimize\", \"Minimized\"" w239 {
          tunnel: w243 -> [w251 w266 w277 w290 w303]
          tunnel: [w253 w267 w279 w292 w305] -> w242
          tunnel: w240 -> [w252 w264 w278 w291 w304]
          frame "Open", "Standard", Default {
            w246 = T4."Standard" ("State")
            n108 = property class="VI"(reference=w252, error in=w251) -> (reference out=w249:refnum<vi>, error out=w250:errorcluster, "FP.State"=w248:T4)
            n109 = Not Equal?(x=w248, y=w246) -> (x != y?=w247:bool)
            n110 = case shown="True" w247 {
              tunnel: [w257 w259] -> w253
              tunnel: w250 -> [w256 w259]
              tunnel: w249 -> [w255 _]
              tunnel: w246 -> [w254 _]
              frame True {
                n111 = invoke class="VI" method="FP.Open"(reference=w255, error in=w256, "Activate"=TRUE, "State"=w254) -> (error out=w257:errorcluster)  [unwired: 1 in, 4 out]
              }
              frame False {
              }
            }
          }
          frame "Close", "Closed" {
            n112 = property class="VI"(reference=w264, error in=w266) -> (reference out=w263:refnum<vi>, error out=w265:errorcluster, "FP.State"=w261:T4)
            n113 = Not Equal?(x=w261, y=T4."Closed" ("Front Panel Window:State")) -> (x != y?=w260:bool)
            n114 = case shown="True" w260 {
              tunnel: [w268 w271] -> w267
              tunnel: w265 -> [w268 w270]
              tunnel: w263 -> [_ w269]
              frame False {
              }
              frame True {
                n115 = invoke class="VI" method="FP.Close"(reference=w269, error in=w270) -> (error out=w271:errorcluster)  [unwired: 1 in, 2 out]
              }
            }
          }
          frame "Hidden", "Hide" {
            w272 = T4."Hidden" ("State")
            n116 = property class="VI"(reference=w278, error in=w277) -> (reference out=w275:refnum<vi>, error out=w276:errorcluster, "FP.State"=w274:T4)
            n117 = Not Equal?(x=w274, y=w272) -> (x != y?=w273:bool)
            n118 = case shown="True" w273 {
              tunnel: [w283 w284] -> w279
              tunnel: w276 -> [w282 w284]
              tunnel: w275 -> [w281 _]
              tunnel: w272 -> [w280 _]
              frame True {
                n119 = invoke class="VI" method="FP.Open"(reference=w281, error in=w282, "State"=w280) -> (error out=w283:errorcluster)  [unwired: 2 in, 4 out]
              }
              frame False {
              }
            }
          }
          frame "Minimize", "Minimized" {
            w285 = T4."Minimized" ("State")
            n120 = property class="VI"(reference=w291, error in=w290) -> (reference out=w288:refnum<vi>, error out=w289:errorcluster, "FP.State"=w287:T4)
            n121 = Not Equal?(x=w287, y=w285) -> (x != y?=w286:bool)
            n122 = case shown="True" w286 {
              tunnel: [w296 w297] -> w292
              tunnel: w289 -> [w295 w297]
              tunnel: w288 -> [w294 _]
              tunnel: w285 -> [w293 _]
              frame True {
                n123 = invoke class="VI" method="FP.Open"(reference=w294, error in=w295, "State"=w293) -> (error out=w296:errorcluster)  [unwired: 2 in, 4 out]
              }
              frame False {
              }
            }
          }
          frame "Maximize", "Maximized" {
            w298 = T4."Maximized" ("State")
            n124 = property class="VI"(reference=w304, error in=w303) -> (reference out=w301:refnum<vi>, error out=w302:errorcluster, "FP.State"=w300:T4)
            n125 = Not Equal?(x=w300, y=w298) -> (x != y?=w299:bool)
            n126 = case shown="True" w299 {
              tunnel: [w309 w310] -> w305
              tunnel: w302 -> [w308 w310]
              tunnel: w301 -> [w307 _]
              tunnel: w298 -> [w306 _]
              frame True {
                n127 = invoke class="VI" method="FP.Open"(reference=w307, error in=w308, "State"=w306) -> (error out=w309:errorcluster)  [unwired: 2 in, 4 out]
              }
              frame False {
              }
            }
          }
        }
        n128 = call <vilib>:"Add State(s) to Queue__jki_lib_state_machine.vi"("State(s) in (\"\")"=w245) -> ("States Out"=w244:string)  [unwired: 14 in]
      }
      frame "---------- Macro ----------" {
        # "Do not put any code in this frame.\n(It is a separator no-op. You can make a copy of this frame to create a new Macro frame)"
        n129 = call <vilib>:"Add State(s) to Queue__jki_lib_state_machine.vi"("State(s) in (\"\")"=w314) -> ("States Out"=w313:string)  [unwired: 14 in]
      }
      frame "Macro: Initialize" {
        w315 = "Data: Initialize\nInitialize Core Data\nUI: Initialize\nUI: Front Panel State >> Open\nXERYON: Initialize"  # Data: Initialize Initialize Core Data UI: Initialize UI: Front Panel State >> Open XERYON: Initialize
        # "Initialization Macro\n(This is called once, when the VI starts)"
        n130 = call <vilib>:"Add State(s) to Queue__jki_lib_state_machine.vi"("State(s) in Front (\"\")"=w315, "State(s) in (\"\")"=w319) -> ("States Out"=w318:string)  [unwired: 13 in]
      }
      frame "Macro: Exit" {
        # "Exit Macro\n(This is called once, when the VI exits)"
        n131 = Unbundle By Name(w327) -> ("Core.Close Panel on Exit?"=w326:bool)
        n132 = Select(t="UI: Front Panel State >> Close", s=w326, f="") -> (s? t:f=w323:string)
        n133 = call <vilib>:"Add State(s) to Queue__jki_lib_state_machine.vi"("State(s) in Front (\"\")"="XERYON: Close", "State(s) in (\"\")"=w323, "State(s) at Back (\"\")"="Data: Cleanup\nExit") -> ("States Out"=w321:string)  [unwired: 12 in]
        n134 = call <vilib>:"Add State(s) to Queue__jki_lib_state_machine.vi"("State(s) in Front (\"\")"=w321, "State(s) in (\"\")"=w330) -> ("States Out"=w329:string)  [unwired: 13 in]
      }
      frame "---------- XERYON ----------" {
        # "Template Separator\n(You can make a copy of, or modify, this frame)"
        n135 = call <vilib>:"Add State(s) to Queue__jki_lib_state_machine.vi"("State(s) in (\"\")"=w334) -> ("States Out"=w333:string)  [unwired: 14 in]
      }
      frame "XERYON: Initialize" {
        # "rad"
        # "3urad"
        # "#why?"
        # "Axis 1"
        # "Read settings file"
        # "STEP 2: Add the connected axis"
        # "STEP 1: Initialize the controller"
        # "Your code here.\n(You can make a copy of, or modify, this frame)"
        n136 = Unbundle By Name(w338) -> ("Controller"=w337:refnum<class "Controller.lvclass">)
        n137 = call-dynamic "initialize.vi"("error in (no error)"=w335, "Baudrate"="Baudrate", "COM Port"="COM Port", "Controller in"=w337) -> ("error out"=w341:errorcluster, "Controller out"=w340:refnum<class "Controller.lvclass">)  [unwired: 6 in]
        n138 = call-dynamic "AddAxis.vi"("Units"="Working Units", "error in (no error)"=w341, "Encoder Resolution"="Axis Resolution", "Axis Letter"="Axis Letter", "Controller in"=w340) -> ("error out"=w344:errorcluster, "Controller out"=w343:refnum<class "Controller.lvclass">)  [unwired: 5 in]
        n139 = call-dynamic "readSettingsFile.vi"("error in (no error)"=w344, "Controller in"=w343) -> ("error out"=w336:errorcluster, "Controller out"=w339:refnum<class "Controller.lvclass">)  [unwired: 8 in]
        n140 = Bundle By Name(cluster=w338, "Controller"=w339) -> (w349:T6)
        n141 = call <vilib>:"Add State(s) to Queue__jki_lib_state_machine.vi"("State(s) in (\"\")"=w351) -> ("States Out"=w350:string)  [unwired: 14 in]
      }
      frame "XERYON: Read Data" {
        # "Display information for axis 1"
        # "Show data cluster"
        # "This block reads all incoming data\nand distributes it to each axis"
        # "Your code here.\n(You can make a copy of, or modify, this frame)"
        n142 = Unbundle By Name(w356) -> ("Controller"=w362:refnum<class "Controller.lvclass">, "Axis Letter"=w358:string)
        n143 = call-dynamic "receiveData.vi"("error in (no error)"=w359, "Controller in"=w362) -> ("error out"=w364:errorcluster, "Controller out"=w363:refnum<class "Controller.lvclass">)  [unwired: 8 in]
        n144 = call-dynamic "getDataCluster.vi"("error in (no error)"=w364, "Axis Letter"=w358, "Controller in"=w363) -> ("error out"=w368:errorcluster, "Information"=→"Status Info":T2, "Controller out"=w365:refnum<class "Controller.lvclass">)  [unwired: 6 in]
        n145 = call-dynamic "getDposInCurrentUnits.vi"("error in (no error)"=w368, "Axis Letter"=w358, "Controller in"=w365) -> ("error out"=w369:errorcluster, "DPOS In Current Units"=w354:dbl, "Controller out"=w366:refnum<class "Controller.lvclass">)  [unwired: 6 in]
        "Desired Position\n[selected units]" <- w354
        n146 = call-dynamic "getEposInCurrentUnits.vi"("error in (no error)"=w369, "Axis Letter"=w358, "Controller in"=w366) -> ("error out"=w370:errorcluster, "EPOS In Current Units"=w355:dbl, "Controller out"=w367:refnum<class "Controller.lvclass">)  [unwired: 6 in]
        "Encoder position \n[selected units]" <- w355
        n147 = Bundle("DPOS In Current Units"=w354, "EPOS In Current Units"=w355) -> (→"Waveform Chart":T3)  [unwired: 1 in]
        n148 = call-dynamic "getStatusBits.vi"("error in (no error)"=w370, "Axis Letter"=w358, "Controller in"=w367) -> ("error out"=w360:errorcluster, "StatusBits"=→"StatusBits":T1, "Controller out"=w361:refnum<class "Controller.lvclass">)  [unwired: 6 in]
        n149 = Bundle By Name(cluster=w356, "Controller"=w361) -> (w357:T6)
        n150 = call <vilib>:"Add State(s) to Queue__jki_lib_state_machine.vi"("State(s) in (\"\")"=w373) -> ("States Out"=w372:string)  [unwired: 14 in]
      }
      frame "XERYON: Close" {
        # "Template Separator\n(You can make a copy of, or modify, this frame)"
        n151 = Unbundle By Name(w377) -> ("Controller"=w376:refnum<class "Controller.lvclass">)
        n152 = call-dynamic "Close.vi"("error in (no error)"=w374, "Controller in"=w376) -> ("error out"=w375:errorcluster)  [unwired: 8 in, 1 out]
        n153 = call <vilib>:"Add State(s) to Queue__jki_lib_state_machine.vi"("State(s) in (\"\")"=w379) -> ("States Out"=w378:string)  [unwired: 14 in]
      }
    }
  }
  "error out" <- w1
